vi "Benchmarking.Integer to String.vi"() -> ()   [LabVIEW 2016]
uses:
  <vilib>/Platform/TimedLoop/XDataNode/timing_clust.ctl
  <vilib>/Platform/TimedLoop/XDataNode/nitl_modes.ctl
  <vilib>/Platform/TimedLoop/XDataNode/wakeup.ctl
  <vilib>/platform/TimedLoop/XDataNode/XDataNode.xnode
  <vilib>/Platform/TimedLoop/XDataNode/XDNodeRunTimeDep.lvlib
panel:
  in  "Processor":i32=-2
  out "time per iteration 2":dbl format="%.0ps"
  out "value as string 2":string
  out "total time 2":dbl format="%_3ps"
  out "total time":dbl format="%_3ps"
  out "time per iteration":dbl format="%.0ps"
  out "value as string":string
  in  "iterations":i32=1000000 format="%.0p"
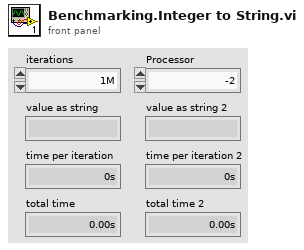
[diagram p1: front panel]
types:
  T1 = typedef "XDNodeRunTimeDep.lvlib/timing_clust.ctl" = cluster{"Expected End [f-1]":u64, "Actual End [f-1]":u64, "Finished Late? [f-1]":bool, "Expected End [i-1]":u64, "Actual End [i-1]":u64, "Finished Late? [i-1]":bool, "Expected Start [i]":u64, "Actual Start [i]":u64, "Expected Start [f]":u64, "Actual Start [f]":u64, "Source Name":string, "Structure Name":string, "Period":i64, "Deadline":i64, "Offset":i64, "Start":i64, "Priority":i32, "Timeout":i32, "Mode":T2, "Wakeup Reason":T3, "Error":errorcluster, "Source Type":string, "Secondary Source Type":string, "Global End Time":u64, "Global Start Time":u64, "Frame Duration":u64, "Iteration Duration":u64, "Assigned CPU":i32, "I/O Scan Engine Mode":u32}
  T2 = typedef "XDNodeRunTimeDep.lvlib/nitl_modes.ctl" = enum32{"No Change", "Process missed periods, maintain original phase", "Discard missed periods, maintain original phase", "Process missed periods, ignore original phase", "Discard missed periods, ignore original phase"}
  T3 = typedef "XDNodeRunTimeDep.lvlib/wakeup.ctl" = enum32{"Normal", "Aborted", "Asynchronous wakeup", "Timing source error", "Timed loop error", "Timeout"}
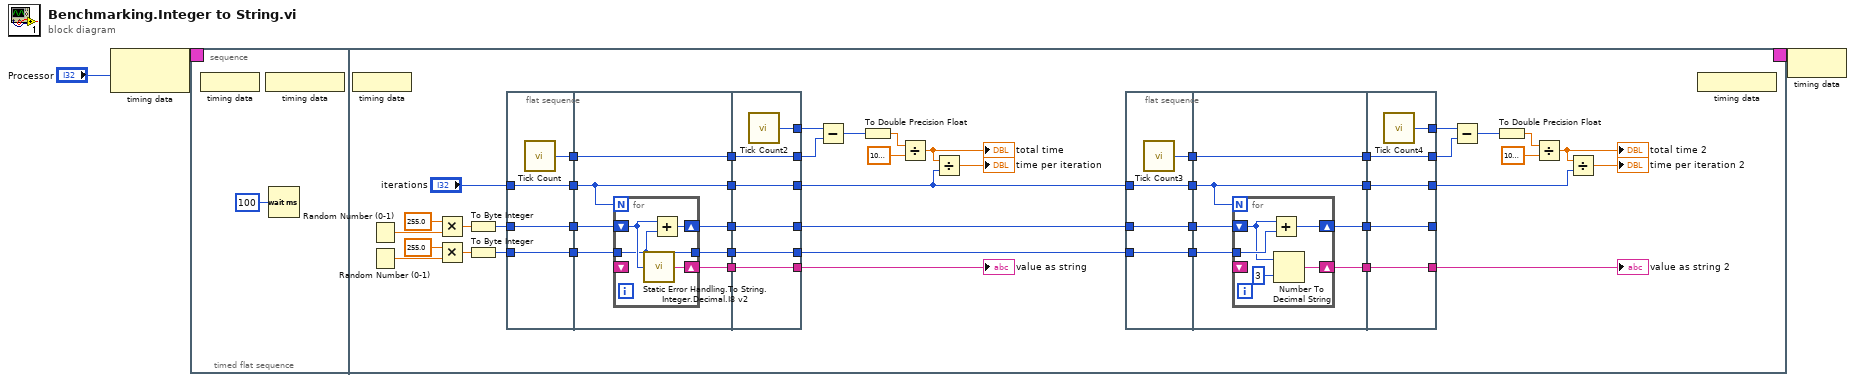
[diagram p0: block diagram]
diagram:
  n1 = node-c288("Processor") -> (w3:T1)
  n2 = timed-sequence {
    timing: w3 -> [_]
    timing-out: [_] -> w2
    n3 = timed-flat-sequence {
      frame #0 {
        n4 = node-c288() -> ()  [unwired: 1 in]
        n5 = node-c288() -> ()  [unwired: 1 out]
        n6 = Wait (ms)(milliseconds to wait=u32 100) -> ()  [unwired: 1 out]
      }
      frame #1 {
        n7 = node-c288() -> ()  [unwired: 1 in]
        n8 = Random Number (0-1)() -> (number: 0 to 1=w35:dbl)
        n9 = Random Number (0-1)() -> (number: 0 to 1=w22:dbl)
        n10 = Multiply(x=255.0, y=w35) -> (x*y=w33:dbl)
        n11 = Multiply(x=255.0, y=w22) -> (x*y=w24:dbl)
        n12 = To Byte Integer(number=w33) -> (8bit integer=w32:i8)
        n13 = To Byte Integer(number=w24) -> (8bit integer=w21:i8)
        n14 = flat-sequence {
          tunnel: "iterations" -> [w75]
          tunnel: w32 -> [w76]
          tunnel: [w76] -> w52
          tunnel: [w75] -> w51
          tunnel: [w74] -> w50
          tunnel: [w73] -> w49
          tunnel: w21 -> [w73]
          tunnel: w52 -> [w83]
          tunnel: w51 -> [w81]
          tunnel: w50 -> [w82]
          tunnel: [w82] -> w48
          tunnel: [w81] -> w47
          tunnel: [w79] -> w46
          tunnel: w49 -> [w80]
          tunnel: [w78] -> w45
          tunnel: [w77] -> w44
          tunnel: w48 -> [w91]
          tunnel: w47 -> [w92]
          tunnel: w46 -> [w93]
          tunnel: [w93] -> w26
          tunnel: [w92] -> w17
          tunnel: [w91] -> w28
          tunnel: [w90] -> w27
          tunnel: w45 -> [w89]
          tunnel: [w89] -> w18
          tunnel: w44 -> [w88]
          tunnel: [w88] -> w16
          frame #0 {
            n15 = call "Tick Count"() -> ("Tick Count(uSec)"=w74:u32)
          }
          frame #1 {
            n16 = for {
              N: w81 -> [_]
              shift-right: [w86] -> w78
              shift-left: w83 -> [w85]
              tunnel: w80 -> [w84]
              shift-right: [w87] -> w79
              shift-left: _ -> [_]
              tunnel: [w84] -> w77
              n17 = call "Static Error Handling.To String.Integer.Decimal.I8 v2.vi"("value"=w85) -> ("value as string"=w87:string)
              n18 = Add(x=w85, y=w84) -> (x+y=w86:i8)
            }
          }
          frame #2 {
            n19 = call "Tick Count2"() -> ("Tick Count(uSec)"=w90:u32)
          }
        }
        n20 = Subtract(x=w27, y=w28) -> (x-y=w20:u32)
        n21 = To Double Precision Float(number=w20) -> (double precision float=w29:dbl)
        n22 = Divide(x=w29, y=1000000.0) -> (x/y=w19:dbl)
        "total time" <- w19
        n23 = Divide(x=w19, y=w17) -> (x/y=→"time per iteration":dbl)
        n24 = flat-sequence {
          tunnel: w17 -> [w55]
          tunnel: w18 -> [w56]
          tunnel: [w56] -> w43
          tunnel: [w55] -> w42
          tunnel: [w54] -> w41
          tunnel: [w53] -> w40
          tunnel: w16 -> [w53]
          tunnel: w43 -> [w62]
          tunnel: w42 -> [w60]
          tunnel: w41 -> [w61]
          tunnel: [w61] -> w39
          tunnel: [w60] -> w38
          tunnel: [w58] -> w37
          tunnel: w40 -> [w59]
          tunnel: [w57] -> w36
          tunnel: w39 -> [w70]
          tunnel: w38 -> [w71]
          tunnel: w37 -> [w72]
          tunnel: [w72] -> w10
          tunnel: [w71] -> w7
          tunnel: [w70] -> w9
          tunnel: [w69] -> w8
          tunnel: w36 -> [w68]
          tunnel: [w68] -> _
          frame #0 {
            n25 = call "Tick Count3"() -> ("Tick Count(uSec)"=w54:u32)
          }
          frame #1 {
            n26 = for {
              N: w60 -> [_]
              shift-right: [w67] -> w57
              shift-left: w62 -> [w65]
              tunnel: w59 -> [w66]
              shift-right: [w64] -> w58
              shift-left: _ -> [_]
              n27 = Add(x=w65, y=w66) -> (x+y=w67:i8)
              n28 = Number To Decimal String(number=w65, width (-)=i16 3) -> (decimal integer string=w64:string)
            }
          }
          frame #2 {
            n29 = call "Tick Count4"() -> ("Tick Count(uSec)"=w69:u32)
          }
        }
        n30 = Subtract(x=w8, y=w9) -> (x-y=w14:u32)
        n31 = To Double Precision Float(number=w14) -> (double precision float=w12:dbl)
        n32 = Divide(x=w12, y=1000000.0) -> (x/y=w15:dbl)
        "total time 2" <- w15
        n33 = Divide(x=w15, y=w7) -> (x/y=→"time per iteration 2":dbl)
        n34 = node-c288() -> ()  [unwired: 1 out]
        "value as string" <- w26
        "value as string 2" <- w10
      }
    }
  }
  n35 = node-c288(w2) -> ()
